vi "camera_selector.vi"(1 "IMAQ interface name":string="img0", 2 "Use external trigger for camera control (IMAQ only)":bool) -> (0 "image acq settings":T2)   [LabVIEW 2010]
uses:
  <vilib>/userDefined/High Color/IMAQdx.ctl
  <vilib>/vision/Avi1.llb/AviRefnum.ctl
  <vilib>/vision/driver/NI_Vision_Acquisition_Software.lvlib
  Image-Stack-Compressor/Stack Reader Wrapper/labview vis/StackReaderWrapper.lvlib
panel:
  out "stack reader handle":u32
  out "Avi Refnum":T3
  out "IMAQ Session Out":refnum<k11>
  in  "AVI/MMF Path":path
  in  "IMAQdx Session":T1="cam0"
  in  "Accept":bool
  in  "Stop":bool
  in  "Image Data Input Source":T4(radio)
  out "error out":errorcluster
  out "IMAQ error":errorcluster
  # "Multi-Worm Tracker \n\n            Image Input Source Selector"
  # "(CameraLink)"
  # "(USB,FireWire, GigE)"
  # "(Pre-recorded)"
  # "(Pre-recorded)"
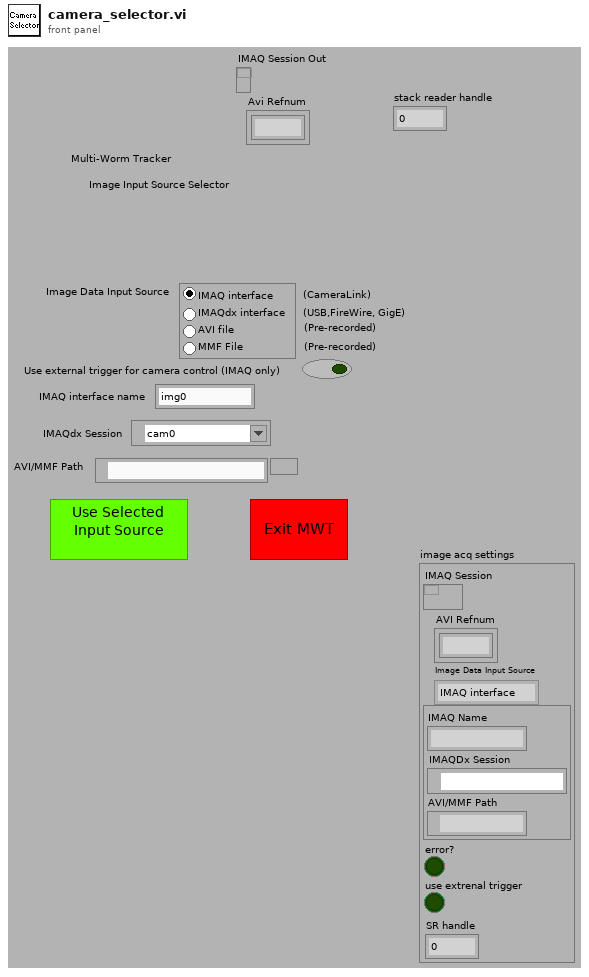
[diagram p1: front panel]
types:
  T1 = typedef "IMAQdx.ctl" = refnum<k21>
  T2 = cluster{"IMAQ Session":refnum<k11>, "AVI Refnum":refnum<k1>, "Image Data Input Source":enum32{"IMAQ interface", "IMAQdx interface", "AVI file", "MMF File"}, cluster{"IMAQ Name":string, "IMAQDx Session":T1, "AVI/MMF Path":path}, "error?":bool, "use extrenal trigger":bool, "SR handle":u32}
  T3 = typedef "AviRefnum.ctl" = refnum<k1>
  T4 = enum32{"IMAQ interface", "IMAQdx interface", "AVI file", "MMF File"}
  T5 = cluster{"Value":string, "Value":refnum<k21>, "Value":path}
  T6 = cluster{"Value":refnum<k11>, "Value":refnum<k1>, "Value":enum32{"IMAQ interface", "IMAQdx interface", "AVI file", "MMF File"}, cluster{"Value":string, "Value":refnum<k21>, "Value":path}, bool, "Value":bool, "Value":u32}
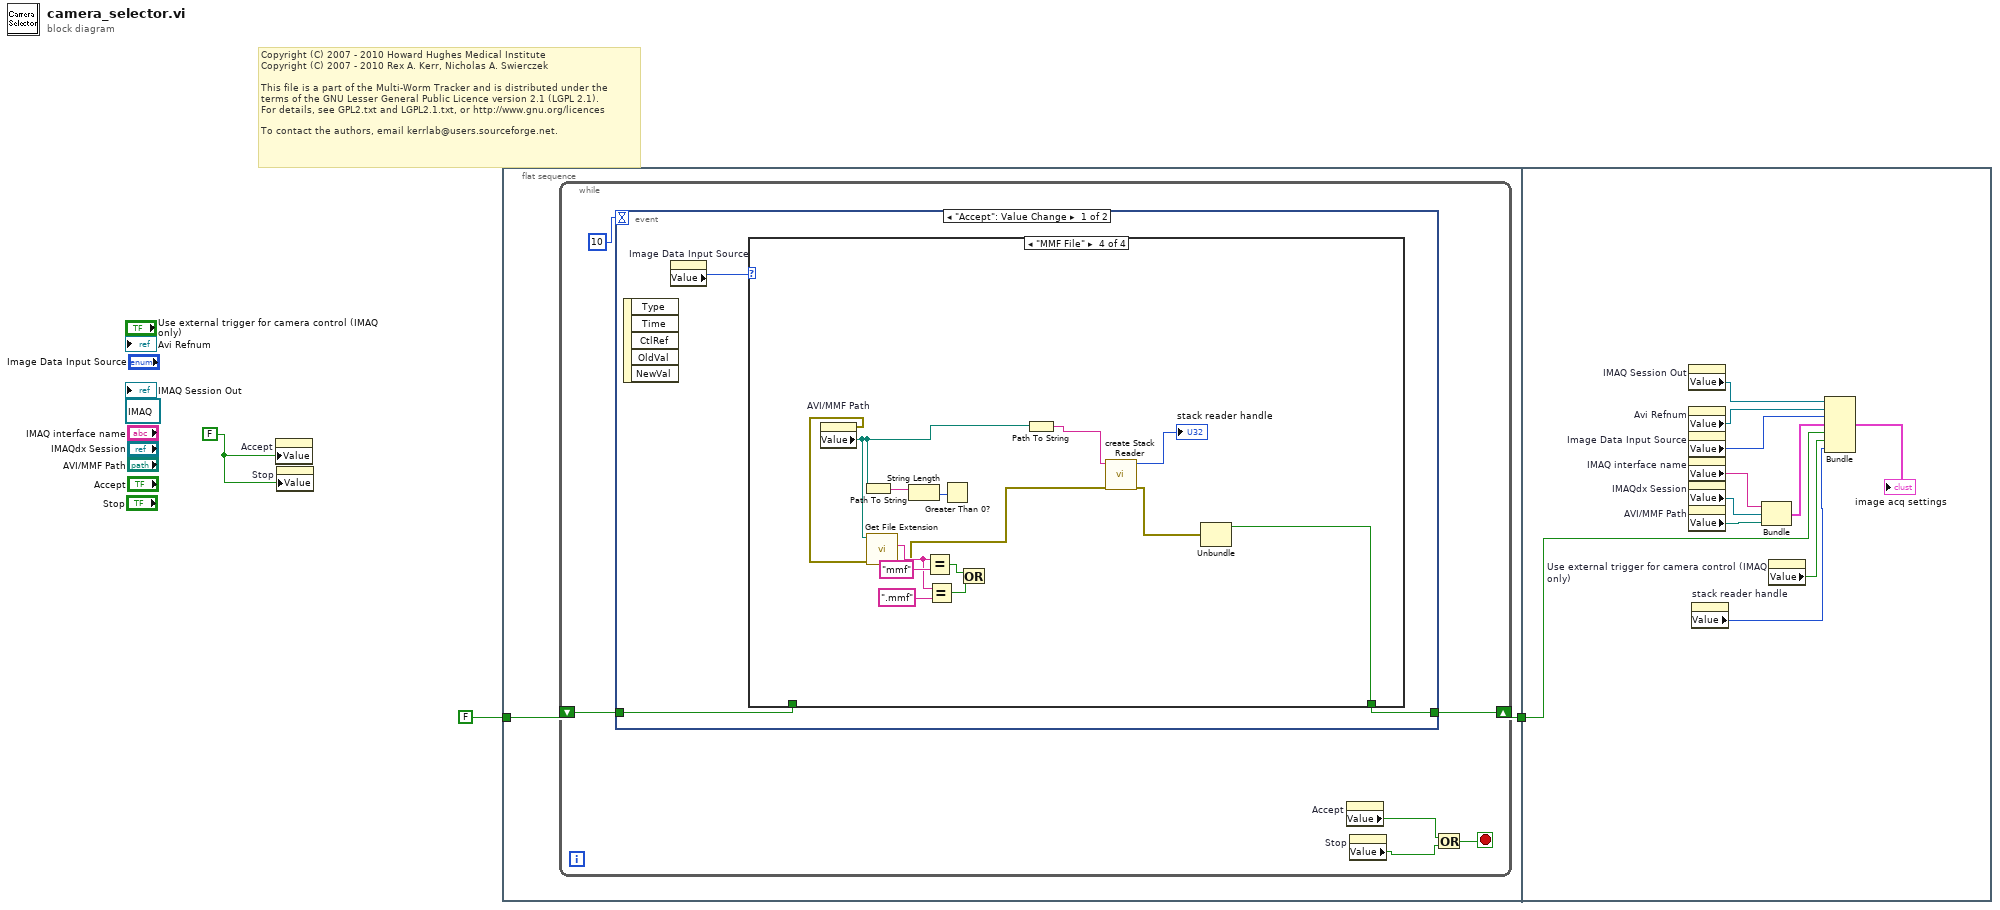
[diagram p0: block diagram]
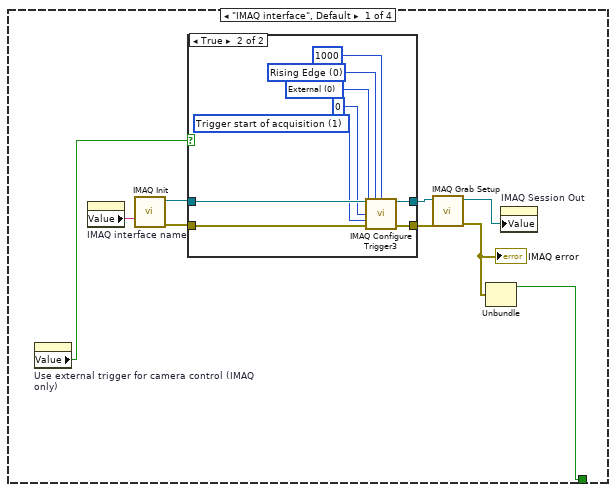
[diagram p2: hidden frame]
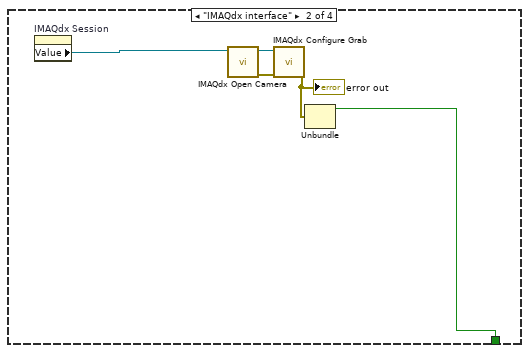
[diagram p4: hidden frame]
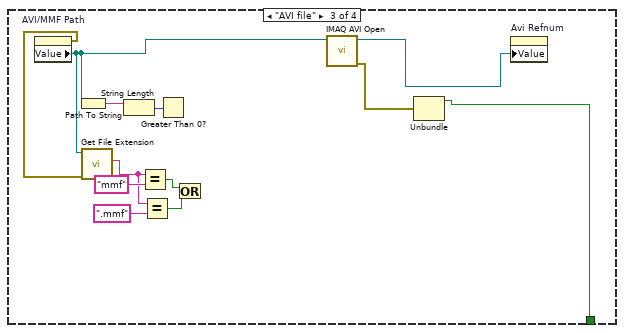
[diagram p5: hidden frame]
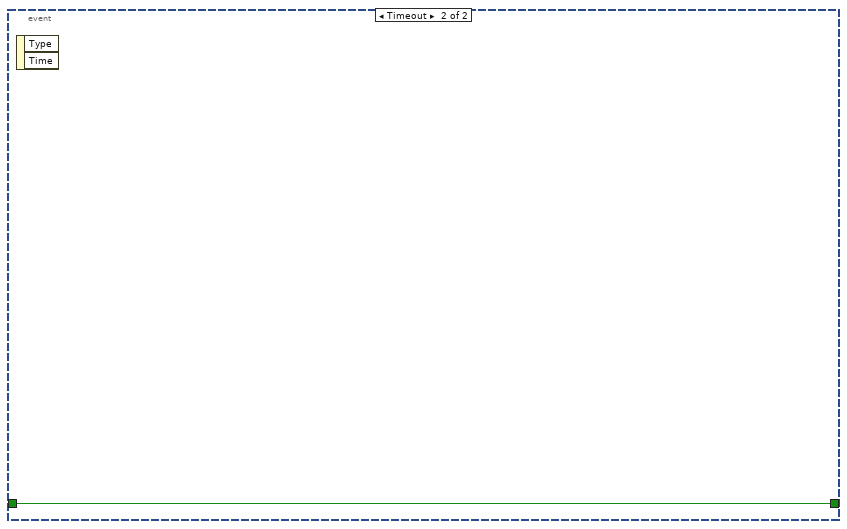
[diagram p6: hidden frame]
diagram:
  w2 = FALSE
  (unwired) refnum<k11> refnum ("IMAQ Session Out")
  # "Copyright (C) 2007 - 2010 Howard Hughes Medical Institute\nCopyright (C) 2007 - 2010 Rex A. Kerr, Nicholas A. Swierczek\n \nThis file is a part of the Multi-Worm Tracker and is distributed under the\nterms of the GNU Lesser General Public Licence version 2.1 (LGPL 2.1).\nFor details, see GPL2.txt and LGPL2.1.txt, or http://www.gnu.org/licences\n \nTo contact the authors, email kerrlab@users.sourceforge.net."
  n1 = property on="Accept" class="Bool (strict)"("Value"=w2) -> ()  [unwired: 2 in, 2 out]
  n2 = property on="Stop" class="Bool (strict)"("Value"=w2) -> ()  [unwired: 2 in, 2 out]
  n3 = flat-sequence {
    tunnel: FALSE -> [w5]
    tunnel: [w4] -> w1
    tunnel: w1 -> [w74]
    frame #0 {
      n4 = while {
        shift-right: [w11] -> w4
        shift-left: w5 -> [w10]
        stop <- w6 stop-if-true
        n5 = event shown="[0] \"Accept\": Value Change" {
          selector: _ -> [_ _]
          dyn-events: _ -> [_ _]
          timeout: 10 -> [_ _]
          tunnel: [w14 w66] -> w11
          tunnel: w10 -> [w13 w66]
          event "Accept": Value Change {
            n6 = event-data() -> ()  [unwired: 1 in, 5 out]
            n7 = property on="Image Data Input Source" class="RadioBtnsControl (strict)"() -> ("Value"=w12:T4)  [unwired: 2 in, 2 out]
            n8 = case shown="\"MMF File\"" w12 {
              tunnel: [w23 w39 w51 w65] -> w14
              tunnel: w13 -> [_ _ _ _]
              frame "IMAQ interface", Default {
                n9 = property on="Use external trigger for camera control (IMAQ only)" class="Bool (strict)"() -> ("Value"=w21:bool)  [unwired: 2 in, 2 out]
                n10 = property on="IMAQ interface name" class="Str"() -> ("Value"=w22:string)  [unwired: 2 in, 2 out]
                n11 = call <vilib>:"IMAQ Init.vi"("Interface Name"=w22) -> ("error out"=w19:errorcluster, "IMAQ Session Out"=w20:refnum<k11>)  [unwired: 9 in]
                n12 = case shown="True" w21 {
                  tunnel: w20 -> [w25 w34]
                  tunnel: [w25 w33] -> w18
                  tunnel: w19 -> [w24 w32]
                  tunnel: [w24 w31] -> w17
                  frame False {
                  }
                  frame True {
                    w26 = u32 1 items=["Disabled", "Trigger start of acquisition", "Trigger start of each buffer list", "Trigger each buffer", "Trigger each line (linescan)", "Trigger end of acquisition"] ("Action")
                    w28 = u32 0 items=["External"=0, "RTSI"=1, "ISO In"=2, "Scaled Encoder"=5, "Software Trigger"=6] ("Type")
                    w29 = u32 0 items=["Rising Edge", "Falling Edge"] ("Polarity")
                    n13 = call <vilib>:"IMAQ Configure Trigger3.vi"("IMAQ Session In"=w34, "Polarity"=w29, "Frame timeout (ms)"=u32 1000, "Type"=w28, "Line Number"=u32 0, "Action"=w26, "error in (no error)"=w32) -> ("IMAQ Session Out"=w33:refnum<k11>, "error out"=w31:errorcluster)  [unwired: 7 in]
                  }
                }
                n14 = call <vilib>:"IMAQ Grab Setup.vi"("error in (no error)"=w17, "IMAQ Session In"=w18) -> ("error out"=w15:errorcluster, "IMAQ Session Out"=w16:refnum<k11>)  [unwired: 8 in]
                "IMAQ error" <- w15
                n15 = Unbundle(w15) -> ("status"=w23:bool)  [unwired: 2 out]
                n16 = property on="IMAQ Session Out" class="Ref (strict)"("Value"=w16) -> ()  [unwired: 2 in, 2 out]
              }
              frame "IMAQdx interface" {
                n17 = property on="IMAQdx Session" class="IMAQdx (strict)"() -> ("Value"=w35:refnum<k21>)  [unwired: 2 in, 2 out]
                n18 = call <vilib>:"IMAQdx Open Camera.vi"("Session In"=w35) -> ("error out"=w38:errorcluster, "Session Out"=w37:T1)  [unwired: 9 in]
                n19 = call <vilib>:"IMAQdx Configure Grab.vi"("error in"=w38, "Session In"=w37) -> ("error out"=w36:errorcluster)  [unwired: 8 in, 1 out]
                "error out" <- w36
                n20 = Unbundle(w36) -> ("status"=w39:bool)  [unwired: 2 out]
              }
              frame "AVI file" {
                n21 = property on="AVI/MMF Path" class="Path"() -> (error out=w42:errorcluster, "Value"=w48:path)  [unwired: 2 in, 1 out]
                n22 = Path To String(path=w48) -> (string=w50:string)
                n23 = call <vilib>:"Get File Extension.vi"("error in (no error)"=w42, "file"=w48) -> ("lowercase file extension"=w46:string)  [unwired: 6 in, 3 out]
                n24 = String Length(string=w50) -> (length=w49:i32)
                n25 = Equal?(x=w46, y="mmf") -> (x = y?=w44:bool)
                n26 = Equal?(x=w46, y=".mmf") -> (x = y?=w43:bool)
                n27 = Greater Than 0?(x=w49) -> ()  [unwired: 1 out]
                n28 = Or(x=w44, y=w43) -> ()  [unwired: 1 out]
                n29 = call "IMAQ AVI Open"("AVI Path"=w48) -> ("error out"=w40:errorcluster, "Avi Refnum"=w41:T3)  [unwired: 9 in]
                n30 = Unbundle(w40) -> ("status"=w51:bool)  [unwired: 2 out]
                n31 = property on="Avi Refnum" class="TypRef (strict)"("Value"=w41) -> ()  [unwired: 2 in, 2 out]
              }
              frame "MMF File" {
                n32 = property on="AVI/MMF Path" class="Path"() -> (error out=w56:errorcluster, "Value"=w62:path)  [unwired: 2 in, 1 out]
                n33 = Path To String(path=w62) -> (string=w64:string)
                n34 = call <vilib>:"Get File Extension.vi"("error in (no error)"=w56, "file"=w62) -> ("error out"=w55:errorcluster, "lowercase file extension"=w60:string)  [unwired: 6 in, 2 out]
                n35 = String Length(string=w64) -> (length=w63:i32)
                n36 = Equal?(x=w60, y="mmf") -> (x = y?=w58:bool)
                n37 = Equal?(x=w60, y=".mmf") -> (x = y?=w57:bool)
                n38 = Greater Than 0?(x=w63) -> ()  [unwired: 1 out]
                n39 = Or(x=w58, y=w57) -> ()  [unwired: 1 out]
                n40 = Path To String(path=w62) -> (string=w54:string)
                n41 = call "create Stack Reader.vi"("error in (no error)"=w55, "fname"=w54) -> ("error out"=w52:errorcluster, "function return"=→"stack reader handle":u32)  [unwired: 8 in]
                n42 = Unbundle(w52) -> ("status"=w65:bool)  [unwired: 2 out]
              }
            }
          }
          event Timeout {
            n43 = event-data() -> ()  [unwired: 1 in, 2 out]
          }
        }
        n44 = property on="Accept" class="Bool (strict)"() -> ("Value"=w9:bool)  [unwired: 2 in, 2 out]
        n45 = property on="Stop" class="Bool (strict)"() -> ("Value"=w8:bool)  [unwired: 2 in, 2 out]
        n46 = Or(x=w9, y=w8) -> (x .or. y?=w6:bool)
      }
    }
    frame #1 {
      n47 = property on="IMAQ Session Out" class="Ref (strict)"() -> ("Value"=w71:refnum<k11>)  [unwired: 2 in, 2 out]
      n48 = property on="Avi Refnum" class="TypRef (strict)"() -> ("Value"=w70:refnum<k1>)  [unwired: 2 in, 2 out]
      n49 = property on="Image Data Input Source" class="RadioBtnsControl (strict)"() -> ("Value"=w77:T4)  [unwired: 2 in, 2 out]
      n50 = property on="IMAQ interface name" class="Str"() -> ("Value"=w76:string)  [unwired: 2 in, 2 out]
      n51 = property on="IMAQdx Session" class="IMAQdx (strict)"() -> ("Value"=w72:refnum<k21>)  [unwired: 2 in, 2 out]
      n52 = property on="AVI/MMF Path" class="Path"() -> ("Value"=w73:path)  [unwired: 2 in, 2 out]
      n53 = property on="stack reader handle" class="DigNum (strict)"() -> ("Value"=w68:u32)  [unwired: 2 in, 2 out]
      n54 = Bundle("Value"=w76, "Value"=w72, "Value"=w73) -> (w75:T5)  [unwired: 1 in]
      n55 = property on="Use external trigger for camera control (IMAQ only)" class="Bool (strict)"() -> ("Value"=w69:bool)  [unwired: 2 in, 2 out]
      n56 = Bundle("Value"=w71, "Value"=w70, "Value"=w77, w75, w74, "Value"=w69, "Value"=w68) -> (→"image acq settings":T6)  [unwired: 1 in]
    }
  }
